vi "624WPI_I2CWrite.vi"(8 "error in (no error)":errorcluster, 9 "I2CDataToSend":u8[](array[numeric]), 10 "I2CRegister":u8, 11 "I2CDevRef":T1={"DevStatus"={"status"=FALSE, "code"=0, "source"=""}, "Controller"=enum."Controller 1", "Device Address"=0, "Handle"=0, "I2C Bus"=enum."Invalid"} {"Device Address" format="%.0x"}) -> (0 "error out":errorcluster, 3 "I2CDevRef":T1={"DevStatus"={"status"=FALSE, "code"=0, "source"=""}, "Controller"=enum."Controller 1", "Device Address"=0, "Handle"=0, "I2C Bus"=enum."Invalid"} {"Device Address" format="%.0x"})   [LabVIEW 2014]
doc: "Writes a byte to the I2C sensor you specify.\n\nThis software is licensed. Open the labview\\readme\\WPI Robotics Library Open Source License.txt file for more information."
uses:
  <vilib>/Rock Robotics/WPI/I2C/WPI_I2CDevRef.ctl
  <vilib>/Rock Robotics/SystemInterfaces/Typedef/FPGA_TypedefDigitalModule.ctl
  <vilib>/Rock Robotics/SystemInterfaces/i2clib/i2c_bus.ctl
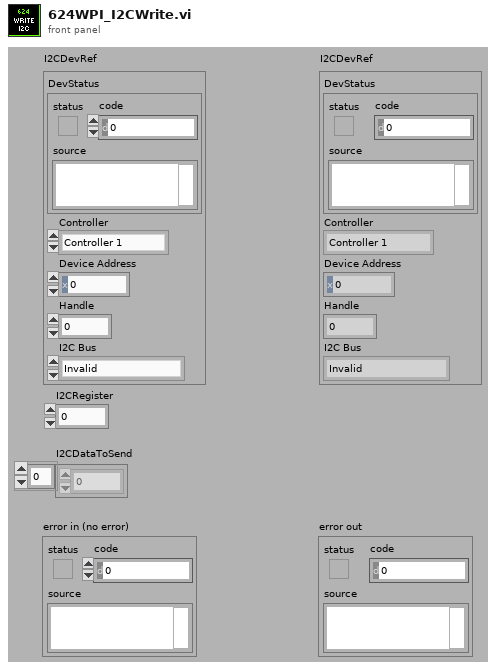
[diagram p1: front panel]
types:
  T1 = typedef "WPI_I2CDevRef.ctl" = cluster{"DevStatus":errorcluster, "Controller":T2, "Device Address":u8, "Handle":i32, "I2C Bus":T3}
  T2 = typedef "FPGA_TypedefDigitalModule.ctl" = enum16{"Controller 1"}
  T3 = typedef "i2c_bus.ctl" = enum16{"I2C On-Board", "I2C MXP", "Invalid"}
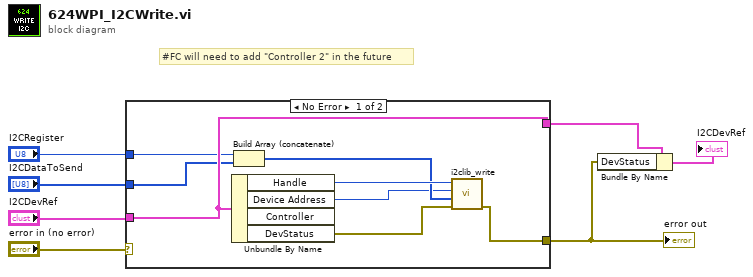
[diagram p0: block diagram]
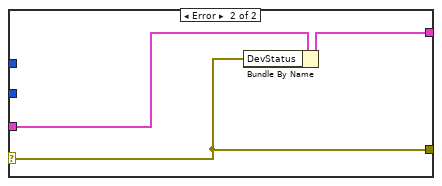
[diagram p2: hidden frame]
diagram:
  # "#FC will need to add \"Controller 2\" in the future"
  n1 = case shown="No Error" "error in (no error)" {
    selector: "error in (no error)" -> [_ w16]
    tunnel: [w8 w16] -> w2
    tunnel: "I2CDevRef" -> [w15 w18]
    tunnel: [w15 w17] -> w3
    tunnel: "I2CRegister" -> [w14 _]
    tunnel: "I2CDataToSend" -> [w13 _]
    frame No Error {
      n2 = Unbundle By Name(w15) -> ("Handle"=w12:i32, "Device Address"=w9:u8, "DevStatus"=w11:errorcluster)  [unwired: 1 out]
      n3 = Build Array (concatenate)(w14, w13) -> (w10:u8[])
      n4 = call <vilib>:"i2clib_write.vi"("error in (no error)"=w11, "send_data"=w10, "dev_addr"=w9, "I2C Reference"=w12) -> ("error out"=w8:errorcluster)  [unwired: 6 in, 1 out]
    }
    frame Error {
      n5 = Bundle By Name(cluster=w18, "DevStatus"=w16) -> (w17:T1)
    }
  }
  "error out" <- w2
  n6 = Bundle By Name(cluster=w3, "DevStatus"=w2) -> (→"I2CDevRef":T1)
